vi "MDAQ_DataWriter.vi"(8 "error in":errorcluster, 9 "Control Cluster":T2 {"CV"."Temperature Array" scale=0.0..100.0}, 10 "Status_Cluster":T1 {"GATESTOP" format="%04x"; "GATESTRT" format="%04x"; "AMPLITUDE" format="%04x"; "M_CYCLES" format="%04x"; "N_CYCLES" format="%04x"; "STEP" format="%04x"; "BASE" format="%04x"; "CHAN" format="%04x"}, 11 "FileRef In":refnum<file>) -> (0 "error out":errorcluster, 3 "refnum out":refnum<file>)   [LabVIEW 2021]
uses:
  GUI_Def.ctl
  Mode_Enum.ctl
  Status_Cluster.ctl
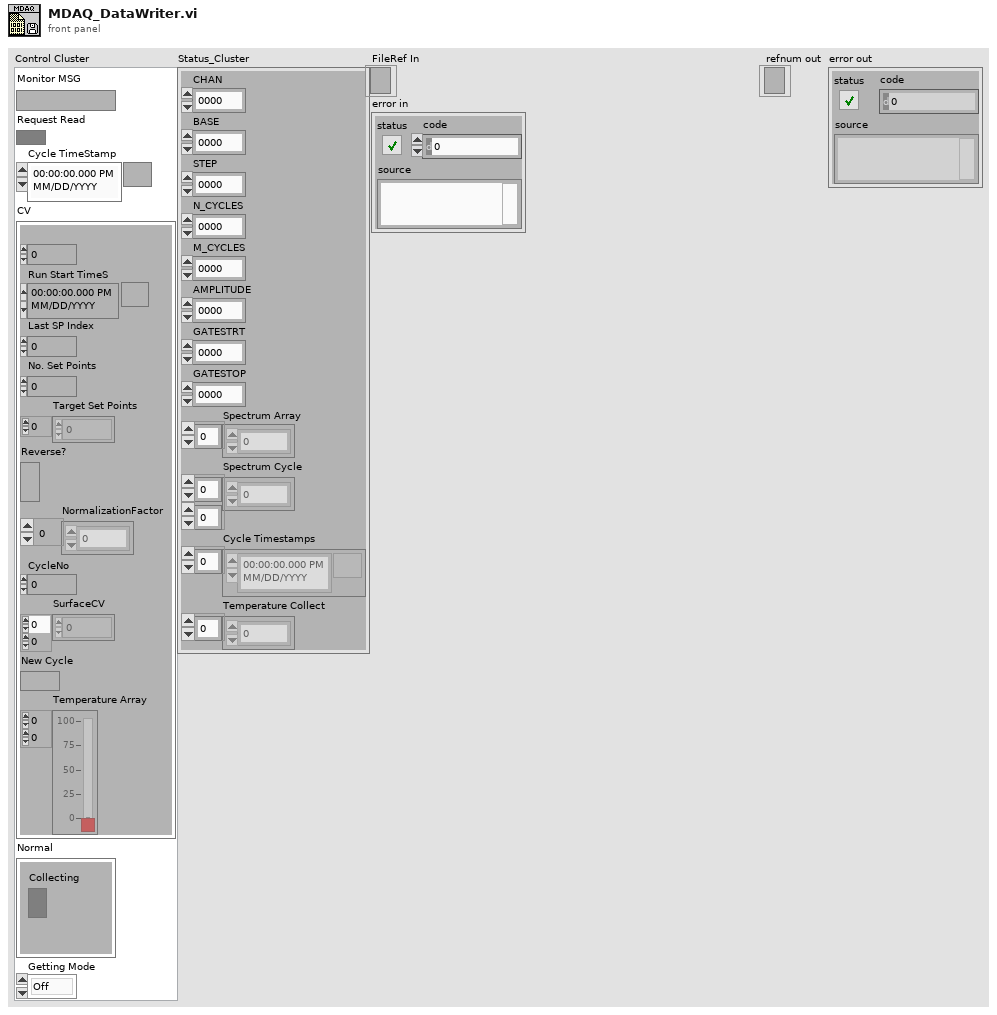
[diagram p1: front panel]
types:
  T1 = typedef "Status_Cluster.ctl" = cluster{"CHAN":u32, "BASE":u32, "STEP":u32, "N_CYCLES":u32, "M_CYCLES":u32, "AMPLITUDE":u32, "GATESTRT":u32, "GATESTOP":u32, "Spectrum Array":u32[], "Spectrum Cycle":u32[][], "Cycle Timestamps":timestamp[], "Temperature Collect":dbl[]}
  T2 = typedef "GUI_Def.ctl" = cluster{"Monitor MSG":string, "Request Read":bool, "Cycle TimeStamp":timestamp, "CV":cluster{"Set Point Index":u32, "Run Start TimeS":timestamp, "Last SP Index":u32, "No. Set Points":u32, "Target Set Points":i32[], "Reverse?":bool, "NormalizationFactor":i32[], "CycleNo":i32, "SurfaceCV":dbl[][], "New Cycle":bool, "Temperature Array":dbl[][]}, "Normal":cluster{"Collecting":bool}, "Getting Mode":T3}
  T3 = typedef "Mode_Enum.ctl" = enum16{"Off", "Normal", "CV+Temp", "CV"}
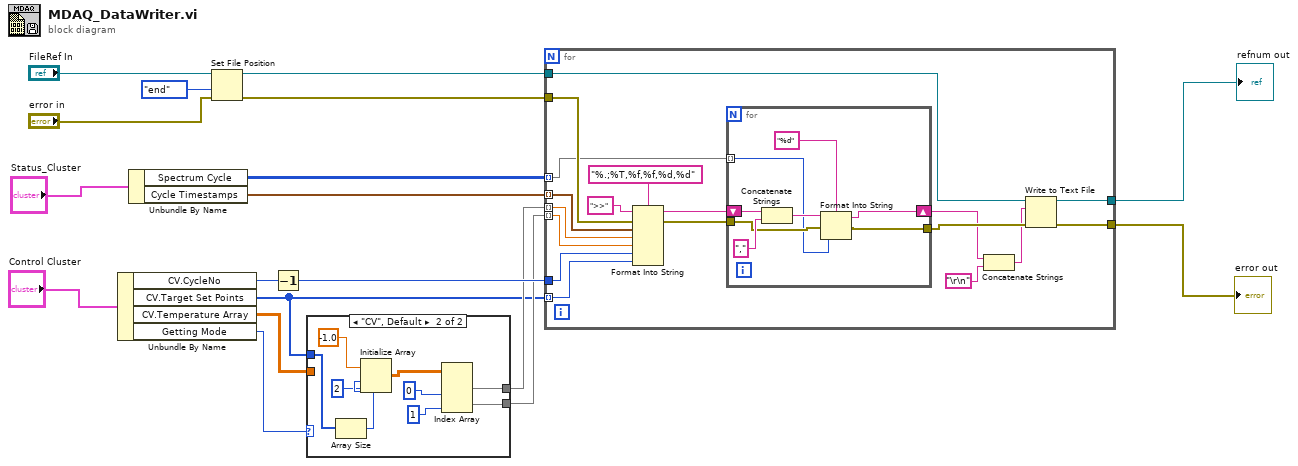
[diagram p0: block diagram]
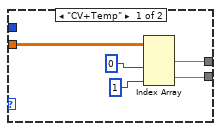
[diagram p2: hidden frame]
diagram:
  n1 = Unbundle By Name("Control Cluster") -> ("CV.CycleNo"=w11:i32, "CV.Target Set Points"=w1:i32[], "CV.Temperature Array"=w4:dbl[][], "Getting Mode"=w5:T3)
  n2 = Unbundle By Name("Status_Cluster") -> ("Spectrum Cycle"=w13:u32[][], "Cycle Timestamps"=w12:timestamp[])
  n3 = Set File Position(refnum="FileRef In", from (0:start)=enum16{"start", "end", "current"}."end", error in="error in") -> (refnum out=w9:refnum<file>, error out=w8:errorcluster)  [unwired: 1 in]
  n4 = Decrement(x=w11) -> (x-1=w10:i32)
  n5 = case shown="\"CV\", Default" w5 {
    tunnel: w4 -> [w23 _]
    tunnel: [w22 w32] -> w3
    tunnel: [w21 w31] -> w2
    tunnel: w1 -> [_ w27]
    frame "CV+Temp" {
      n6 = Index Array(array=w23, index (col) #1=0 ("index (row)"), index (col) #2=1 ("index (row)")) -> (element #1=w22:dbl[], element #2=w21:dbl[])  [unwired: 2 in]
    }
    frame "CV", Default {
      n7 = Array Size(array=w27) -> (size(s)=w26:i32)
      n8 = Initialize Array(-1.0 ("element"), w26, 2 ("dimension size")) -> (w24:dbl[][])
      n9 = Index Array(array=w24, index (col) #1=0 ("index (row)"), index (col) #2=1 ("index (row)")) -> (element #1=w32:dbl[], element #2=w31:dbl[])  [unwired: 2 in]
    }
  }
  n10 = for {
    tunnel: w13 -> [w42] mode=indexing
    tunnel: w12 -> [w48] mode=indexing
    tunnel: w10 -> [w45]
    tunnel: w1 -> [w44] mode=indexing
    tunnel: w9 -> [w39]
    tunnel: w8 -> [w50]
    tunnel: w3 -> [w47] mode=indexing
    tunnel: w2 -> [w46] mode=indexing
    tunnel: [w34] -> w7
    tunnel: [w33] -> w6
    n11 = Format Into String(format string="%.;%T,%f,%f,%d,%d", initial string=">>", error in=w50, w48, w47, w46, w45, w44) -> (resulting string=w41:string, error out=w40:errorcluster)
    n12 = for {
      tunnel: w42 -> [w54] mode=indexing
      tunnel: w40 -> [w55]
      shift-right: [w52] -> w37
      shift-left: w41 -> [w58]
      tunnel: [w51] -> w38
      n13 = Concatenate Strings(w58, ",") -> (w56:string)
      n14 = Format Into String(format string="%d", initial string=w56, error in=w55, w54) -> (resulting string=w52:string, error out=w51:errorcluster)
    }
    n15 = Concatenate Strings(w37, "\r\n") -> (w36:string)
    n16 = Write to Text File(file (use dialog)=w39, text=w36, error in=w38) -> (refnum out=w34:refnum<file>, error out=w33:errorcluster)  [unwired: 1 in, 1 out]
  }
  "refnum out" <- w7
  "error out" <- w6
